vi "Calculate Triangle Illumination.vi"(6 "Fill Colour":u32(colorbox)=12517256, 7 "Light Direction":T1, 11 "Triangle Normal":T1) -> (3 "Fill Colour Actual":u32(colorbox)=12517256)   [LabVIEW 2020, in "3D.lvlib"]
uses:
  3D.lvlib
  Vector 3D.ctl
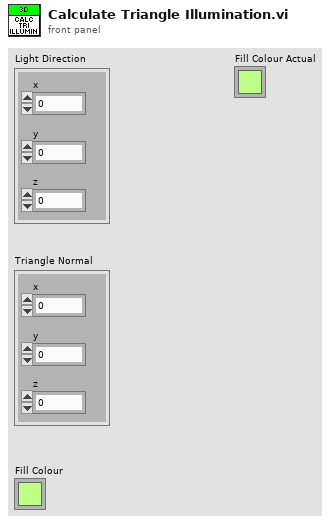
[diagram p1: front panel]
types:
  T1 = typedef "3D.lvlib/Vector 3D.ctl" = cluster{"x":sgl, "y":sgl, "z":sgl}
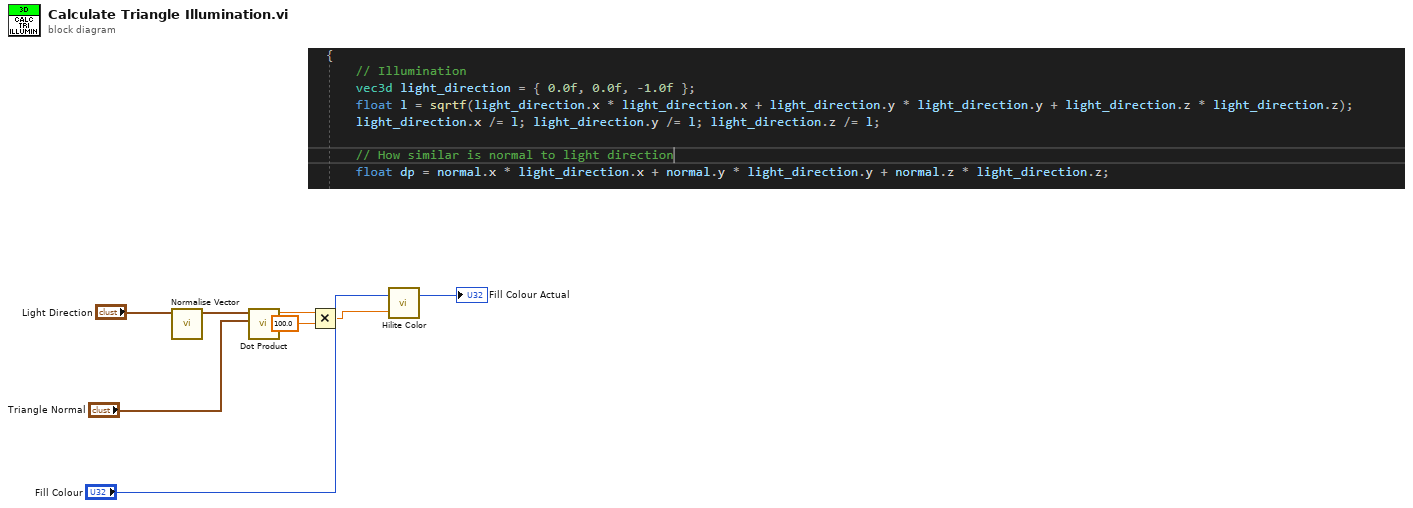
[diagram p0: block diagram]
diagram:
  n1 = call "Normalise Vector.vi"("Vector 3D"="Light Direction") -> ("Vector 3D Normalised"=w7:T1)  [unwired: 10 in]
  n2 = call "Dot Product.vi"("Vector B"="Triangle Normal", "Vector A"=w7) -> ("Dot Product"=w4:sgl)  [unwired: 9 in]
  n3 = Multiply(x=w4, y=sgl 100.0) -> (x*y=w2:sgl)
  n4 = call <vilib>:"Hilite Color.vi"("Percentage(30)"=w2, "Color In"="Fill Colour") -> ("Hilite"=→"Fill Colour Actual":u32)  [unwired: 1 out]
